vi "in range_by_percent.vi"(8 "error in (no error)":errorcluster, 9 "setpoint":dbl, 10 "tol %":dbl, 11 "x":dbl) -> (0 "error out":errorcluster, 1 "lower limit":dbl, 2 "In Range?":bool, 3 "upper limit":dbl)   [LabVIEW 2020]
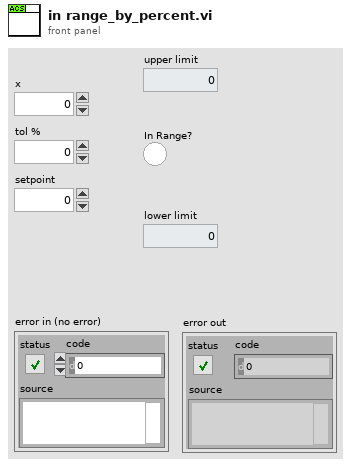
[diagram p1: front panel]
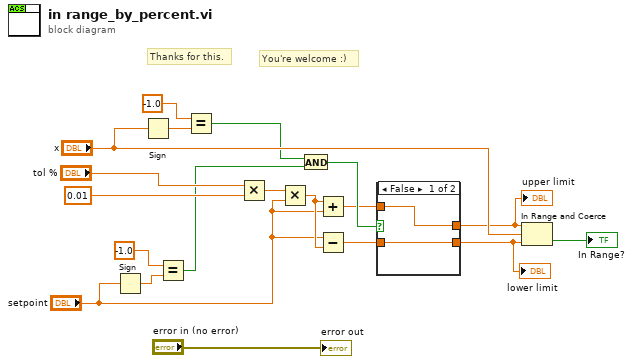
[diagram p0: block diagram]
diagram:
  # "You're welcome :)"
  # "Thanks for this."
  n1 = Sign(1:"setpoint") -> (0:w10:dbl)
  n2 = Sign(1:"x") -> (0:w12:dbl)
  n3 = Equal?(x=-1.0, y=w10) -> (x = y?=w7:bool)
  n4 = Equal?(x=-1.0, y=w12) -> (x = y?=w6:bool)
  n5 = Multiply(x="tol %", y=0.01) -> (x*y=w17:dbl)
  n6 = Multiply(x=w17, y="setpoint") -> (x*y=w16:dbl)
  n7 = And(x=w6, y=w7) -> (x .and. y?=w5:bool)
  n8 = Add(x=w16, y="setpoint") -> (x+y=w4:dbl)
  n9 = Subtract(x="setpoint", y=w16) -> (x-y=w2:dbl)
  n10 = case shown="False" w5 {
    tunnel: w4 -> [w21 w23]
    tunnel: [w21 w22] -> w3
    tunnel: w2 -> [w20 w22]
    tunnel: [w20 w23] -> w1
    frame False {
    }
    frame True {
    }
  }
  "upper limit" <- w3
  "lower limit" <- w1
  n11 = In Range and Coerce(upper limit=w3, x="x", lower limit=w1) -> (In Range?=→"In Range?":bool)  [unwired: 1 out]
  "error out" <- "error in (no error)"
